vi "ZCAN_Receive.vi"(4 "error in (no error)":errorcluster caption="错误输入（无错误）", 7 "can_handle":u32) -> (0 "error out":errorcluster caption="错误输出", 1 "CANFD数据帧数组":T1(array[cluster]), 2 "CAN数据帧数组":T2(array[cluster]), 3 "Receive_Num":u32)   [LabVIEW 2020, in "zlgcan.lvlib"]
uses:
  zlgcan.lvlib
  bin/zlgcan_wrap.dll
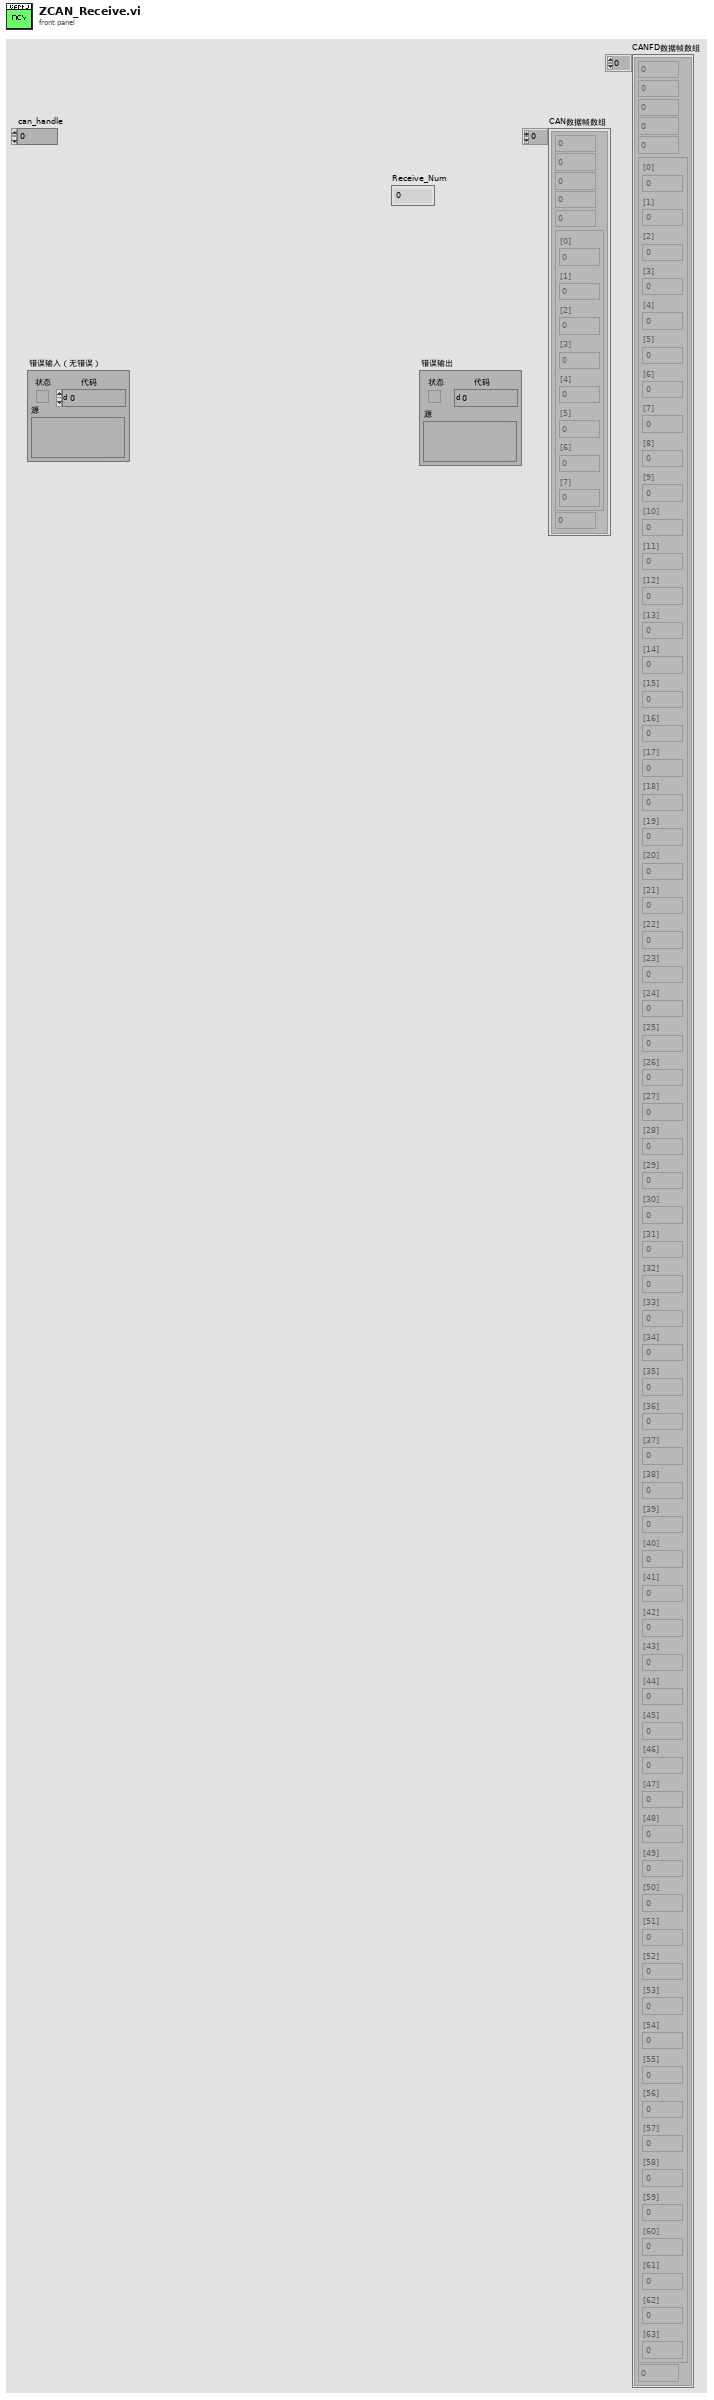
[diagram p1: front panel]
types:
  T1 = cluster{u32, u8, u8, u8, u8, cluster{"[0]":u8, "[1]":u8, "[2]":u8, "[3]":u8, "[4]":u8, "[5]":u8, "[6]":u8, "[7]":u8, "[8]":u8, "[9]":u8, "[10]":u8, "[11]":u8, "[12]":u8, "[13]":u8, "[14]":u8, "[15]":u8, "[16]":u8, "[17]":u8, "[18]":u8, "[19]":u8, "[20]":u8, "[21]":u8, "[22]":u8, "[23]":u8, "[24]":u8, "[25]":u8, "[26]":u8, "[27]":u8, "[28]":u8, "[29]":u8, "[30]":u8, "[31]":u8, "[32]":u8, "[33]":u8, "[34]":u8, "[35]":u8, "[36]":u8, "[37]":u8, "[38]":u8, "[39]":u8, "[40]":u8, "[41]":u8, "[42]":u8, "[43]":u8, "[44]":u8, "[45]":u8, "[46]":u8, "[47]":u8, "[48]":u8, "[49]":u8, "[50]":u8, "[51]":u8, "[52]":u8, "[53]":u8, "[54]":u8, "[55]":u8, "[56]":u8, "[57]":u8, "[58]":u8, "[59]":u8, "[60]":u8, "[61]":u8, "[62]":u8, "[63]":u8}, u64}[]
  T2 = cluster{u32, u8, u8, u8, u8, cluster{"[0]":u8, "[1]":u8, "[2]":u8, "[3]":u8, "[4]":u8, "[5]":u8, "[6]":u8, "[7]":u8}, u64}[]
  T3 = cluster{"[0]":u8, "[1]":u8, "[2]":u8, "[3]":u8, "[4]":u8, "[5]":u8, "[6]":u8, "[7]":u8, "[8]":u8, "[9]":u8, "[10]":u8, "[11]":u8, "[12]":u8, "[13]":u8, "[14]":u8, "[15]":u8, "[16]":u8, "[17]":u8, "[18]":u8, "[19]":u8, "[20]":u8, "[21]":u8, "[22]":u8, "[23]":u8, "[24]":u8, "[25]":u8, "[26]":u8, "[27]":u8, "[28]":u8, "[29]":u8, "[30]":u8, "[31]":u8, "[32]":u8, "[33]":u8, "[34]":u8, "[35]":u8, "[36]":u8, "[37]":u8, "[38]":u8, "[39]":u8, "[40]":u8, "[41]":u8, "[42]":u8, "[43]":u8, "[44]":u8, "[45]":u8, "[46]":u8, "[47]":u8, "[48]":u8, "[49]":u8, "[50]":u8, "[51]":u8, "[52]":u8, "[53]":u8, "[54]":u8, "[55]":u8, "[56]":u8, "[57]":u8, "[58]":u8, "[59]":u8, "[60]":u8, "[61]":u8, "[62]":u8, "[63]":u8}
  T4 = cluster{u32, u8, u8, u8, u8, cluster{"[0]":u8, "[1]":u8, "[2]":u8, "[3]":u8, "[4]":u8, "[5]":u8, "[6]":u8, "[7]":u8, "[8]":u8, "[9]":u8, "[10]":u8, "[11]":u8, "[12]":u8, "[13]":u8, "[14]":u8, "[15]":u8, "[16]":u8, "[17]":u8, "[18]":u8, "[19]":u8, "[20]":u8, "[21]":u8, "[22]":u8, "[23]":u8, "[24]":u8, "[25]":u8, "[26]":u8, "[27]":u8, "[28]":u8, "[29]":u8, "[30]":u8, "[31]":u8, "[32]":u8, "[33]":u8, "[34]":u8, "[35]":u8, "[36]":u8, "[37]":u8, "[38]":u8, "[39]":u8, "[40]":u8, "[41]":u8, "[42]":u8, "[43]":u8, "[44]":u8, "[45]":u8, "[46]":u8, "[47]":u8, "[48]":u8, "[49]":u8, "[50]":u8, "[51]":u8, "[52]":u8, "[53]":u8, "[54]":u8, "[55]":u8, "[56]":u8, "[57]":u8, "[58]":u8, "[59]":u8, "[60]":u8, "[61]":u8, "[62]":u8, "[63]":u8}, u64}
  T5 = cluster{"[0]":u8, "[1]":u8, "[2]":u8, "[3]":u8, "[4]":u8, "[5]":u8, "[6]":u8, "[7]":u8}
  T6 = cluster{u32, u8, u8, u8, u8, cluster{"[0]":u8, "[1]":u8, "[2]":u8, "[3]":u8, "[4]":u8, "[5]":u8, "[6]":u8, "[7]":u8}, u64}
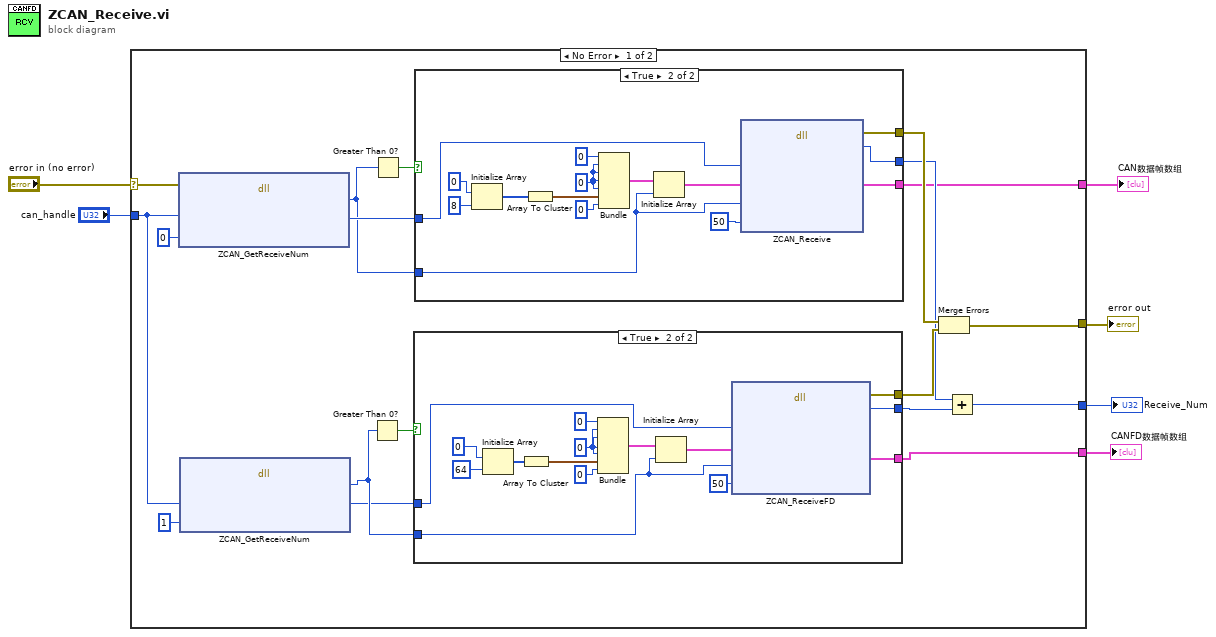
[diagram p0: block diagram]
diagram:
  n1 = case shown="No Error" "error in (no error)" {
    selector: "error in (no error)" -> [w24 w55]
    tunnel: [w13 w55] -> w5
    tunnel: "can_handle" -> [w18 _]
    tunnel: [w10 _] -> w3
    tunnel: [w9 _] -> w2
    tunnel: [w8 _] -> w1
    frame No Error {
      n2 = dll-call lib="E:/Jabil tools/JabilTestLib/ZLG_CANFD/bin/zlgcan_wrap.dll" fn="ZCAN_GetReceiveNum"(error in=w24, "通道句柄"=w18, "协议"=u8 0) -> ("缓冲区帧数"=w21:u32, "通道句柄"=w22:u32)  [unwired: 3 in, 2 out]
      n3 = dll-call lib="E:/Jabil tools/JabilTestLib/ZLG_CANFD/bin/zlgcan_wrap.dll" fn="ZCAN_GetReceiveNum"("通道句柄"=w18, "协议"=u8 1) -> ("缓冲区帧数"=w16:u32, "通道句柄"=w7:u32)  [unwired: 4 in, 2 out]
      n4 = Greater Than 0?(x=w16) -> (x > 0?=w17:bool)
      n5 = Greater Than 0?(x=w21) -> (x > 0?=w23:bool)
      n6 = case shown="True" w17 {
        tunnel: w16 -> [_ w28]
        tunnel: [_ w38] -> w8
        tunnel: [_ w37] -> w14
        tunnel: [_ w25] -> w12
        tunnel: w7 -> [_ w26]
        frame False {
        }
        frame True {
          w32 = u8 0
          n7 = Initialize Array(u8 0 ("元素"), u32 64 ("维数大小")) -> (w34:u8[])
          n8 = Array To Cluster(array=w34) -> (cluster=w35:T3)
          n9 = Bundle(u32 0, w32, w32, w32, w32, w35, u64 0) -> (w36:T4)  [unwired: 1 in]
          n10 = Initialize Array(w36, w28) -> (w27:T1)
          n11 = dll-call lib="E:/Jabil tools/JabilTestLib/ZLG_CANFD/bin/zlgcan_wrap.dll" fn="ZCAN_ReceiveFD"("通道句柄"=w26, "数据帧数组"=w27, "数据帧数"=w28, "超时时间"=50) -> (error out=w37:errorcluster, "已接收帧数"=w25:u32, "数据帧数组"=w38:T1)  [unwired: 6 in, 1 out]
        }
      }
      n12 = case shown="True" w23 {
        tunnel: w22 -> [_ w44]
        tunnel: w21 -> [_ w43]
        tunnel: [_ w42] -> w9
        tunnel: [_ w41] -> w15
        tunnel: [_ w40] -> w11
        frame False {
        }
        frame True {
          w50 = u8 0
          n13 = Initialize Array(u8 0 ("元素"), u32 8 ("维数大小")) -> (w52:u8[])
          n14 = Array To Cluster(array=w52) -> (cluster=w53:T5)
          n15 = Bundle(u32 0, w50, w50, w50, w50, w53, u64 0) -> (w54:T6)  [unwired: 1 in]
          n16 = Initialize Array(w54, w43) -> (w45:T2)
          n17 = dll-call lib="E:/Jabil tools/JabilTestLib/ZLG_CANFD/bin/zlgcan_wrap.dll" fn="ZCAN_Receive"("通道句柄"=w44, "数据帧数组"=w45, "数据帧数"=w43, "超时时间"=50) -> (error out=w41:errorcluster, "已接收帧数"=w40:u32, "数据帧数组"=w42:T2)  [unwired: 6 in, 1 out]
        }
      }
      n18 = Merge Errors(w15, w14) -> (w13:errorcluster)
      n19 = Add(x=w11, y=w12) -> (x+y=w10:u32)
    }
    frame Error {
    }
  }
  "error out" <- w5
  "Receive_Num" <- w3
  "CAN数据帧数组" <- w2
  "CANFD数据帧数组" <- w1
